vi "EventLog.Filter.vi"(0 "data in":T3[](array[typedef]) {"ts" format="%<%X\n%x>T"}, 1 "Event.Sets":T1 {"dtm_End" format="%<%.1X\n%x>T"; "dtm_Begin" format="%<%.1X\n%x>T"}) -> (2 "data out":T3[](array[typedef]) {"ts" format="%<%X\n%x>T"})   [LabVIEW 2016]
uses:
  EventLog.EventGui.ctl
  EventLog.EventLevel.ctl
  EventLog.EventSource.ctl
  Translator/Translator.Message.ctl
  EventLog.Gui.Sets.ctl
  EventLog.EventLevelOperatorGui.ctl
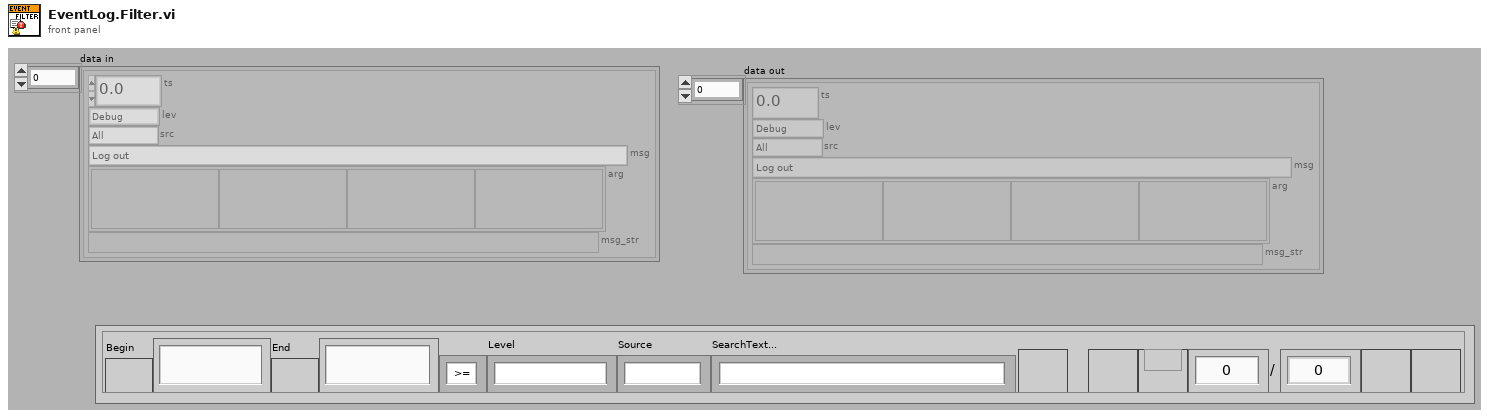
[diagram p1: front panel]
types:
  T1 = typedef "EventLog.Gui.Sets.ctl" = cluster{"IncludeBegin":bool, "dtm_Begin":timestamp, "IncludeEnd":bool, "dtm_End":timestamp, "Events Level Operator":T2, "Level":u16, "Source":u16, "SearchText":string, "Refresh":bool, "Pages":i32, "PageNo":i32, "First":bool, "Prev":bool, "Next":bool, "Last":bool}
  T2 = typedef "EventLog.EventLevelOperatorGui.ctl" = enum16{">=", "=", "<="}
  T3 = typedef "EventLog.EventGui.ctl" = cluster{"ts":dbl, "lev":T4, "src":T5, "msg":T6, "arg":variant[], "msg_str":string}
  T4 = typedef "EventLog.EventLevel.ctl" = enum8{"Debug", "Info", "Warning", "Error"}
  T5 = typedef "EventLog.EventSource.ctl" = enum16{"All", "Gui", "Cache", "PLC1", "PLC2", "PLC3", "DB", "DB01", "DB02", "DB03", "DB04", "DB05", "DB06", "DB07", "DB08", "DB09", "DB10", "DB11", "DB12", "DB13", "DB14", "DB15", "DB16"}
  T6 = typedef "Translator.Message.ctl" = enum16{"-", "Event confirmed", "Log out", "Log in", "Shutdown", "Cancel", "Start", "Continue", "Stop", "On", "Off", "OK", "NOK", "NOK %s", "This", "Prev", "Home", "Work", "In progress...", "Missing", "Empty", "Hardware failure", "Initial", "Error %d >> %s", "Error %d >> %s >> %s", "Starting %s", "Quitting %s", "Configured", "Initializing", "Quitting", "Loading", "Running %s", "Stopped", "Summary", "Do you want to continue?", "Do you want to exit?", "Log out?", "System", "All", "IDLE", "Translating...%s", "Not found", "Alarm %s", "Run", "Skip", "Abort", "Repeat", "Please wait...", "Database disconnected", "Login to database successful", "Login to database failed: %d; %s", "Get process step data for %s", "Changeover off", "Changeover into %s", "Product %s | %s found in cache with status %d at previous station", "Product %s | %s found in database with status %d at previous station", "Product %s | %s not found in cache at previous station", "Product %s | %s not found in database at previous station", "Product %s | %s found in cache with status %d at this station (%d repetion)", "Product %s | %s found in database with status %d at this station (%d repetition)", "Product %s | %s not found in cache at this station", "Product %s | %s not found in database at this station", "Product %s | %s found in cache for component %s | %s", "Product %s | %s found in database for component %s | %s", "Product not found in cache for component %s | %s", "Product not found in database for component %s | %s", "Product %s | %s connected with component %s | %s (cache)", "Product %s | %s connected with component %s | %s (database)", "New data for %s | %s (cache)", "New data for %s | %s (database)", "File %s moved (cache)", "File %s deleted (cache)", "Msg %d >> %s", "PLC LifeBit Failure", "Reconnecting DB", "Reconnecting PLC", "Free disk space is below 1GB - contact technician"}
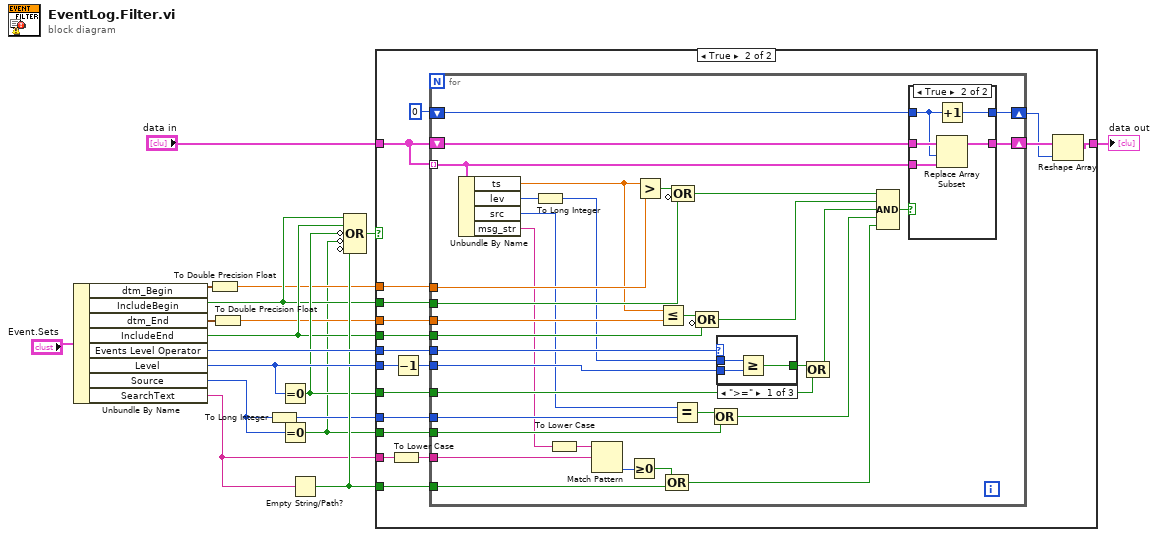
[diagram p0: block diagram]
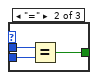
[diagram p4: hidden frame]
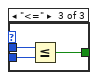
[diagram p5: hidden frame]
diagram:
  n1 = Unbundle By Name("Event.Sets") -> ("dtm_Begin"=w18:timestamp, "IncludeBegin"=w9:bool, "dtm_End"=w17:timestamp, "IncludeEnd"=w10:bool, "Events Level Operator"=w16:T2, "Level"=w13:u16, "Source"=w2:u16, "SearchText"=w7:string)
  n2 = To Double Precision Float(number=w18) -> (double precision float=w5:dbl)
  n3 = To Double Precision Float(number=w17) -> (double precision float=w4:dbl)
  n4 = To Long Integer(number=w2) -> (32bit integer=w3:i32)
  n5 = Equal To 0?(x=w13) -> (x = 0?=w11:bool)
  n6 = Equal To 0?(x=w2) -> (x = 0?=w1:bool)
  n7 = Empty String/Path?(string/path=w7) -> (empty?=w12:bool)
  n8 = Compound Arithmetic op=OR(w9, w10, invert w11, invert w1, invert w12) -> (w8:bool)
  n9 = case shown="True" w8 {
    tunnel: w5 -> [_ w37]
    tunnel: w9 -> [_ w36]
    tunnel: w4 -> [_ w35]
    tunnel: w10 -> [_ w34]
    tunnel: w16 -> [_ w33]
    tunnel: w11 -> [_ w32]
    tunnel: [w19 w28] -> w15
    tunnel: "data in" -> [w19 w27]
    tunnel: w13 -> [_ w26]
    tunnel: w7 -> [_ w24]
    tunnel: w12 -> [_ w23]
    tunnel: w3 -> [_ w20]
    tunnel: w1 -> [_ w21]
    frame False {
    }
    frame True {
      n10 = To Lower Case(string=w24) -> (all lower case string=w25:string)
      n11 = Decrement(x=w26) -> (x-1=w22:u16)
      n12 = for {
        tunnel: w27 -> [w38] mode=indexing
        tunnel: w37 -> [w71]
        tunnel: w36 -> [w70]
        tunnel: w35 -> [w68]
        tunnel: w34 -> [w66]
        tunnel: w33 -> [w64]
        tunnel: w22 -> [w61]
        tunnel: w32 -> [w62]
        shift-right: [w55] -> w30
        shift-left: w27 -> [w56]
        shift-right: [w52] -> w29
        shift-left: 0 -> [w53]
        tunnel: w25 -> [w51]
        tunnel: w23 -> [w47]
        tunnel: w20 -> [w43]
        tunnel: w21 -> [w44]
        n13 = Unbundle By Name(w38) -> ("ts"=w65:dbl, "lev"=w63:T4, "src"=w41:T5, "msg_str"=w42:string)
        n14 = To Long Integer(number=w63) -> (32bit integer=w60:i32)
        n15 = To Lower Case(string=w42) -> (all lower case string=w46:string)
        n16 = Match Pattern(string=w46, regular expression=w51) -> (offset past match=w49:i32)  [unwired: 1 in, 3 out]
        n17 = Greater Or Equal To 0?(x=w49) -> (x >= 0?=w48:bool)
        n18 = Greater?(x=w65, y=w71) -> (0:w69:bool)
        n19 = Less Or Equal?(x=w65, y=w68) -> (x <= y?=w67:bool)
        n20 = Compound Arithmetic op=OR(w48, w47) -> (w50:bool)
        n21 = Compound Arithmetic op=OR(w69, invert w70) -> (w57:bool)
        n22 = Equal?(x=w41, y=w43) -> (x = y?=w40:bool)
        n23 = Compound Arithmetic op=OR(w67, invert w66) -> (w58:bool)
        n24 = Compound Arithmetic op=OR(w40, w44) -> (w39:bool)
        n25 = case shown="\">=\"" w64 {
          tunnel: w60 -> [w81 w84 w87]
          tunnel: w61 -> [w80 w83 w86]
          tunnel: [w79 w82 w85] -> w59
          frame ">=" {
            n26 = Greater Or Equal?(x=w81, y=w80) -> (x >= y?=w79:bool)
          }
          frame "=" {
            n27 = Equal?(x=w84, y=w83) -> (x = y?=w82:bool)
          }
          frame "<=" {
            n28 = Less Or Equal?(x=w87, y=w86) -> (x <= y?=w85:bool)
          }
        }
        n29 = Compound Arithmetic op=OR(w59, w62) -> (w45:bool)
        n30 = Compound Arithmetic op=AND(w57, w58, w45, w39, w50) -> (w54:bool)
        n31 = case shown="True" w54 {
          tunnel: w56 -> [w73 w78]
          tunnel: [w73 w77] -> w55
          tunnel: w38 -> [_ w76]
          tunnel: w53 -> [w72 w75]
          tunnel: [w72 w74] -> w52
          frame False {
          }
          frame True {
            n32 = Increment(x=w75) -> (x+1=w74:i32)
            n33 = Replace Array Subset(array=w78, new element=w76, index=w75) -> (w77:T3[])
          }
        }
      }
      n34 = Reshape Array(w30, w29) -> (w28:T3[])
    }
  }
  "data out" <- w15
